vi "john set wavelength.vi"() -> ()   [LabVIEW 2012]
uses:
  Global/GPIB Numbers.vi
panel:
  in  "Set to WL":dbl
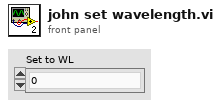
[diagram p1: front panel]
types:
  T1 = typedef "USBCCD Type Def.ctl" = cluster{"Name":string, "Unique ID":string, "Mono Unique ID":string}
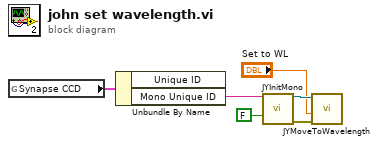
[diagram p0: block diagram]
diagram:
  n1 = global read "GPIB Numbers.vi" "Synapse CCD"() -> (w6:T1)
  n2 = Unbundle By Name(w6) -> ("Mono Unique ID"=w5:string)  [unwired: 1 out]
  n3 = call "JYInitMono.vi"("Unique ID"=w5, "Force Init"=FALSE) -> ("Mono RefNum out"=w3:refnum<k7>, "error out"=w2:errorcluster)  [unwired: 9 in, 3 out]
  n4 = call "JYMoveToWavelength.vi"("error in (no error)"=w2, "Target WL"="Set to WL", "RefNum In"=w3) -> ()  [unwired: 1 in, 3 out]
